vi "Get settings chain.vi"(8 "error in (no error)":errorcluster, 11 "ImageStackBase in":refnum<class "ImageStack.lvclass">) -> (0 "error out":errorcluster, 1 "class name":string[](array[string]), 2 "settings":variant[](array[variant]), 3 "ImageStackBase out":refnum<class "ImageStack.lvclass">)   [LabVIEW 2012, in "ImageStack.lvclass"]
doc: "Returns an array of variants containing the settings clusters of each class in the inheritance chain (lowest child class first), together with an array of all class names in the inheritance chain.\n\nFor classes without settings cluster, the settings chain contains empty variants."
uses:
  ImageStack.lvclass
  <vilib>/Distrio/Murmex/Murmex/Murmex.lvclass
  ImageStack.lvclass/ImageStack.ctl
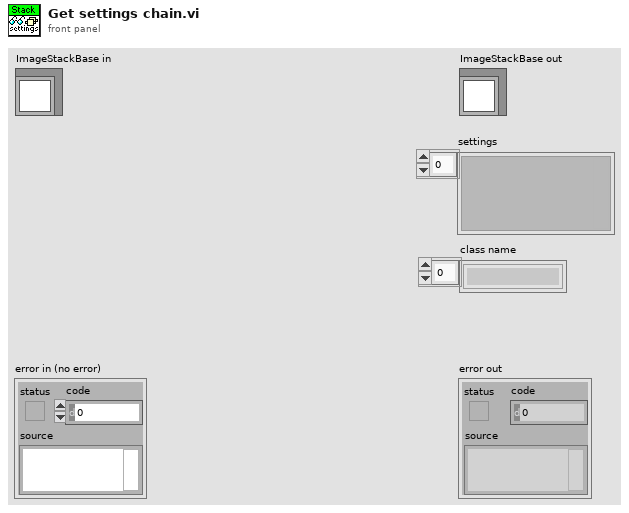
[diagram p1: front panel]
types:
  T1 = typedef "ImageStack.lvclass/settings_cluster.ctl" = cluster{"Number of frames":u16, "Frame rate":dbl[unit], "Step size":dbl[unit], "Subfolder levels":string[], "Translation speed":dbl[unit], "File name":string}
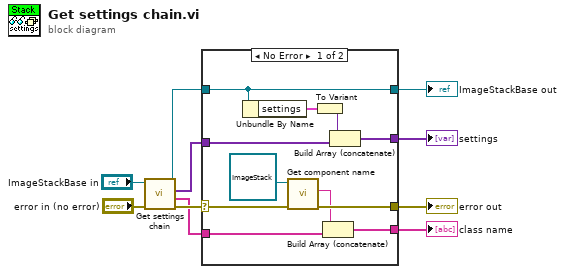
[diagram p0: block diagram]
diagram:
  n1 = call-parent "Get settings chain.vi"("error in (no error)"="error in (no error)", "MurmexBase in"="ImageStackBase in") -> ("error out"=w8:errorcluster, "class name"=w6:string[], "settings"=w4:variant[], "MurmexBase out"=w3:refnum<class "ImageStack.lvclass">)  [unwired: 6 in]
  n2 = case shown="No Error" w8 {
    selector: w8 -> [w21 w24]
    tunnel: [w20 w24] -> w7
    tunnel: w6 -> [w18 w25]
    tunnel: [w16 w25] -> w5
    tunnel: w4 -> [w15 w23]
    tunnel: w3 -> [w14 w22]
    tunnel: [w14 w22] -> w2
    tunnel: [w11 w23] -> w1
    frame No Error {
      n3 = Unbundle By Name(w14) -> ("settings"=w13:T1)
      n4 = call <vilib>:"Get component name.vi"("error in (no error)"=w21, "Murmex in"=refnum<class "ImageStack.lvclass"> refnum ("ImageStack")) -> ("error out"=w20:errorcluster, "component name"=w19:string)  [unwired: 7 in, 1 out]
      n5 = To Variant(anything=w13) -> (Variant=w12:variant)
      n6 = Build Array (concatenate)(w19, w18) -> (w16:string[])
      n7 = Build Array (concatenate)(w12, w15) -> (w11:variant[])
    }
    frame Error {
    }
  }
  "error out" <- w7
  "ImageStackBase out" <- w2
  "settings" <- w1
  "class name" <- w5
